vi "Teleop.vi"(10 "Match Info":T1={"Autonomous Elapsed Seconds"=0.0, "TeleOp Elapsed Seconds"=0.0, "Disabled Elapsed Seconds"=0.0, "Visited Autonomous"=FALSE, "Visited TeleOp"=FALSE, "Visited Disabled"=FALSE, "Autonomous Settings"={"Autonomous Style"=enum."Independent", "VI Refnum"=refnum}}, 11 "Call Context":T2) -> ()   [LabVIEW 2012]
doc: "This VI is called for each TeleOp packet received from the DS where the robot is not disabled. It is often used to read from the joysticks and update I/O or to update setpoints for timed control loops. It should complete and return within 20 milliseconds or it may miss DS packets."
uses:
  <vilib>/Rock Robotics/WPI/DriverStation/WPI_DriverStationDerivedRobotMode.ctl
  <vilib>/Rock Robotics/WPI/DriverStation/WPI_DriverStationMatch Info.ctl
  <vilib>/Rock Robotics/WPI/DriverStation/DriverStationLCD/WPI_DriverStationLCDLCDLine.ctl
  Robot Global Data.vi
  <vilib>/Rock Robotics/WPI/Joystick/WPI_JoystickGetSetRefNum.vi
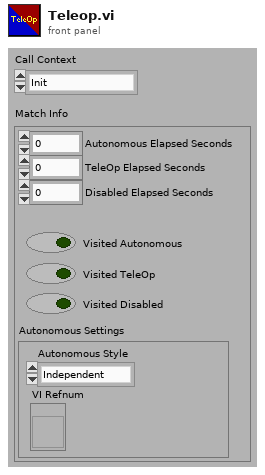
[diagram p1: front panel]
types:
  T1 = typedef "WPI_DriverStationMatch Info.ctl" = cluster{"Autonomous Elapsed Seconds":dbl, "TeleOp Elapsed Seconds":dbl, "Disabled Elapsed Seconds":dbl, "Visited Autonomous":bool, "Visited TeleOp":bool, "Visited Disabled":bool, "Autonomous Settings":cluster{"Autonomous Style":enum16{"Iterative", "Independent"}, "VI Refnum":refnum<vi>}}
  T2 = typedef "WPI_DriverStationDerivedRobotMode.ctl" = enum16{"Init", "Execute", "Stop"}
  T3 = typedef "WPI_DriverStationLCDLCDLine.ctl" = enum16{"Main - Line 1", "User - Line 2", "User - Line 3", "User - Line 4", "User - Line 5", "User - Line 6"}
  T4 = typedef "WPI_MotorControlDeviceRef.ctl" = cluster{"DeviceStatus":errorcluster, "Type":enum16{"PWM", "CAN"}, "PWM":cluster{"Digital Module":T5, "PWM Channel":T6, "DeadBand":T7}, "CAN":cluster{"Device Number":u8, "Control Mode":T8, "Semaphore":T9, "Max Vout":dbl}, "Invert":bool, "TransformRef":T10, "InvTransformRef":T10}
  T5 = typedef "FPGA_TypedefDigitalModule.ctl" = enum16{"Digital Module 1", "Digital Module 2"}
  T6 = typedef "FPGA_DIOPWMChannel.ctl" = enum8{"PWM 1", "PWM 2", "PWM 3", "PWM 4", "PWM 5", "PWM 6", "PWM 7", "PWM 8", "PWM 9", "PWM 10", "Invalid"}
  T7 = typedef "WPI_PWMDeadband.ctl" = cluster{"Name":string, "maxPositivePwm":i32, "minPositivePwm":i32, "centerPwm":i32, "maxNegativePwm":i32, "minNegativePwm":i32, "angularRange":u16}
  T8 = typedef "WPI_CANJaguar_ControlMode.ctl" = enum8{"Percent VBus", "Current", "Speed", "Position", "Voltage"}
  T9 = typedef "Semaphore RefNum" = refnum<k1>
  T10 = typedef "WPI_PWMTransform_ConPane.ctl" = refnum<vi>
  T11 = typedef "WPI_JoystickDevRef.ctl" = cluster{"Device":T12}
  T12 = typedef "WPI_JoystickDeviceEnum.ctl" = enum16{"USB 1", "USB 2", "USB 3", "USB 4", "Kinect 1", "Kinect 2"}
  T13 = typedef "WPI_JoystickButtonState.ctl" = cluster{"Button 1":bool, "Button 2":bool, "Button 3":bool, "Button 4":bool, "Button 5":bool, "Button 6":bool, "Button 7":bool, "Button 8":bool, "Button 9":bool, "Button 10":bool, "Button 11":bool, "Button 12":bool}
  T14 = cluster{"axis 1 (x)":dbl, "axis 2 (y)":dbl, "axis 3 (throttle)":dbl, "axis 4":dbl, "axis 5":dbl, "axis 6":dbl}
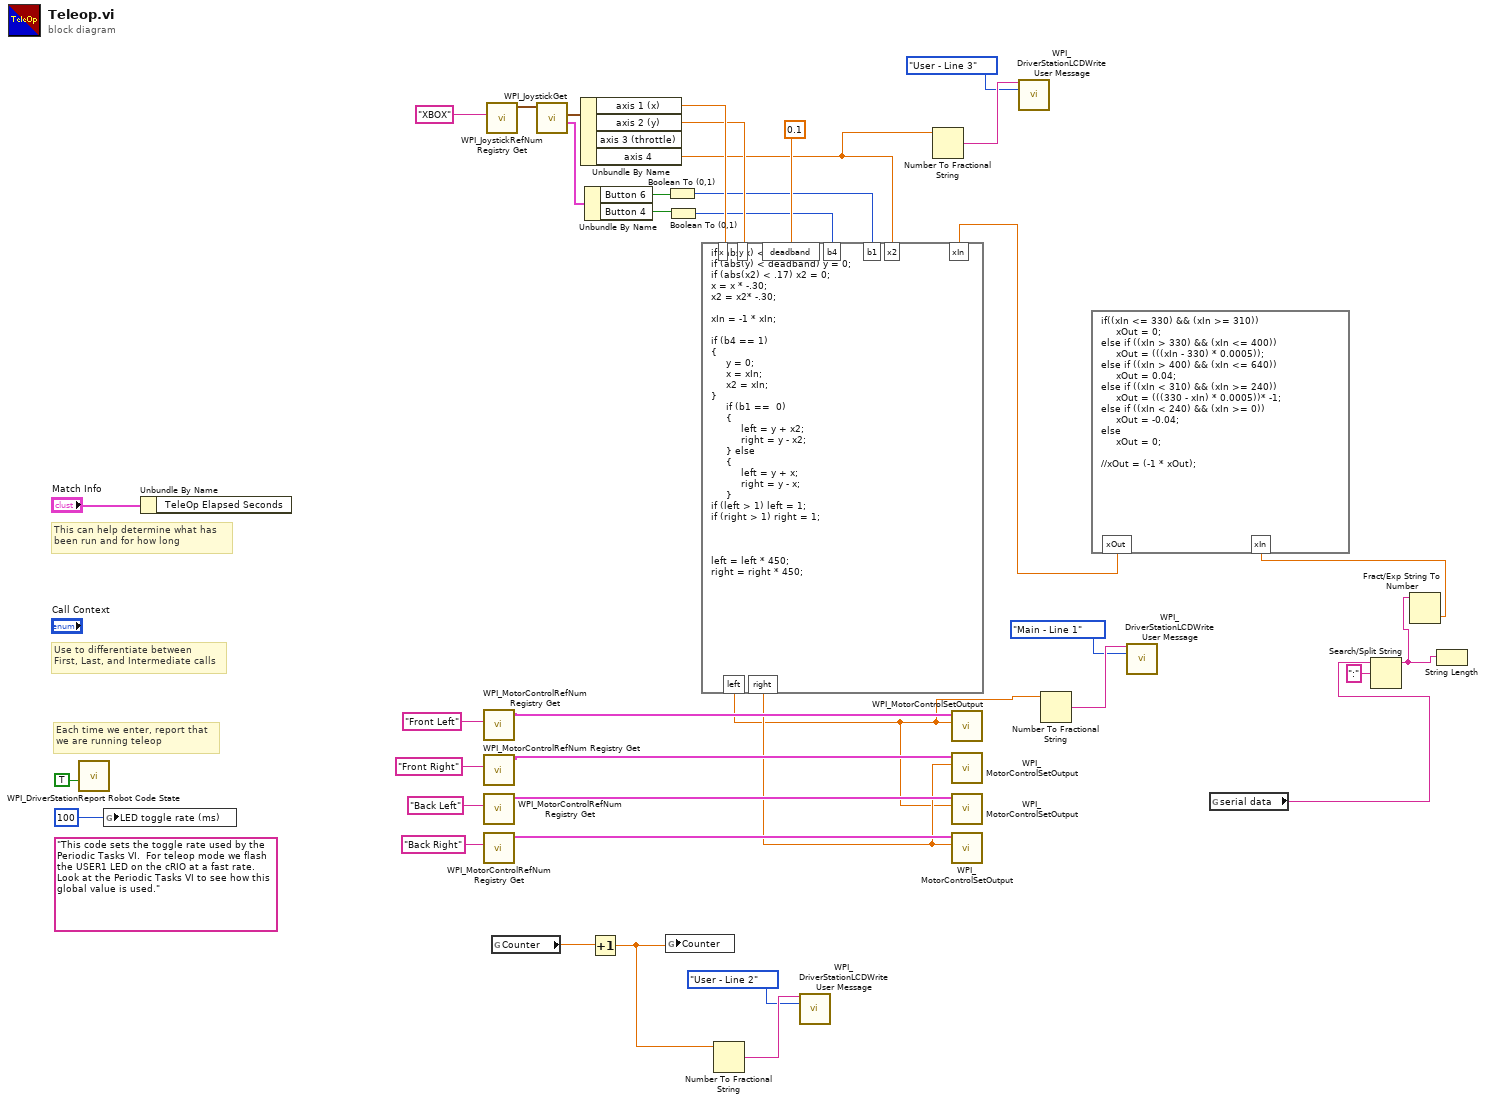
[diagram p0: block diagram]
diagram:
  (unwired) "This code sets the toggle rate used by the Periodic Tasks VI.  For teleop mode we flash the USER1 LED on the cRIO at a fast rate.  Look at the Periodic Tasks VI to see how this global value is used."
  # "Each time we enter, report that\nwe are running teleop"
  # "Use to differentiate between\nFirst, Last, and Intermediate calls"
  # "This can help determine what has\nbeen run and for how long"
  n1 = call <vilib>:"WPI_DriverStationReport Robot Code State.vi"("TeleOp"=TRUE ("Autonomous")) -> ()  [unwired: 10 in, 1 out]
  n2 = global write "Robot Global Data.vi" "LED toggle rate (ms)"(u32 100 ("LED ms toggle rate")) -> ()
  n3 = Unbundle By Name("Match Info") -> ()  [unwired: 1 out]
  n4 = call <vilib>:"WPI_MotorControlRefNum Registry Get.vi"("refnum name"="Front Left") -> ("MotorControlDevRef"=w30:T4)  [unwired: 9 in, 1 out]
  n5 = call <vilib>:"WPI_MotorControlRefNum Registry Get.vi"("refnum name"="Front Right") -> ("MotorControlDevRef"=w29:T4)  [unwired: 9 in, 1 out]
  n6 = call <vilib>:"WPI_MotorControlRefNum Registry Get.vi"("refnum name"="Back Left") -> ("MotorControlDevRef"=w28:T4)  [unwired: 9 in, 1 out]
  n7 = call <vilib>:"WPI_MotorControlRefNum Registry Get.vi"("refnum name"="Back Right") -> ("MotorControlDevRef"=w27:T4)  [unwired: 9 in, 1 out]
  n8 = call <vilib>:"WPI_JoystickRefNum Registry Get.vi"("refnum name"="XBOX") -> ("JoystickDevRef"=w24:T11)  [unwired: 1 in, 9 out]
  n9 = global read "Robot Global Data.vi" "Counter"() -> (w18:dbl)
  n10 = call <vilib>:"WPI_JoystickGet.vi"("JoystickDevRef"=w24) -> ("Buttons"=w11:T13, "Axes"=w23:T14)  [unwired: 1 in, 4 out]
  n11 = Unbundle By Name(w23) -> ("axis 1 (x)"=w22:dbl, "axis 2 (y)"=w12:dbl, "axis 4"=w8:dbl)  [unwired: 1 out]
  n12 = Unbundle By Name(w11) -> ("Button 6"=w10:bool, "Button 4"=w3:bool)
  n13 = Increment(x=w18) -> (x+1=w15:dbl)
  n14 = global write "Robot Global Data.vi" "Counter"(w15) -> ()
  n15 = Boolean To (0,1)(Boolean=w10) -> (0, 1=w9:i16)
  n16 = Boolean To (0,1)(Boolean=w3) -> (0, 1=w2:i16)
  n17 = Number To Fractional String(number=w15) -> (F-format string=w17:string)  [unwired: 3 in]
  n18 = call <vilib>:"WPI_DriverStationLCDWrite User Message.vi"("line text"=w17, "line"=WPI_DriverStationLCDLCDLine."User - Line 2") -> ()  [unwired: 13 in, 1 out]
  n19 = Number To Fractional String(number=w8) -> (F-format string=w14:string)  [unwired: 3 in]
  n20 = call <vilib>:"WPI_DriverStationLCDWrite User Message.vi"("line text"=w14, "line"=WPI_DriverStationLCDLCDLine."User - Line 3") -> ()  [unwired: 13 in, 1 out]
  n21 = global read "Robot Global Data.vi" "serial data"() -> (w1:string)
  n22 = Search/Split String(string=w1, search string/char (-)=":") -> (substring before match=w6:string)  [unwired: 1 in, 2 out]
  n23 = Fract/Exp String To Number(string=w6) -> (number=w5:dbl)  [unwired: 3 in, 1 out]
  n24 = formula code="if((xIn <= 330) && (xIn >= 310))\n     xOut = 0;\nelse if ((xIn > 330) && (xIn <= 400))\n     xOut = (((xIn - 330) * 0.0005));\nelse if ((xIn > 400) && (xIn <= 640))\n     xOut = 0.04;\nelse if ((xIn < 310) && (xIn >= 240))\n     xOut = (((330 - xIn) * 0.0005))* -1;\nelse if ((xIn < 240) && (xIn >= 0))\n     xOut = -0.04;\nelse\n     xOut = 0;\n\n//xOut = (-1 * xOut);"("xIn"=w5) -> ("xOut"=w4:dbl)
  n25 = formula code="if (abs(x) < .17) x = 0;\nif (abs(y) < deadband) y = 0;\nif (abs(x2) < .17) x2 = 0;\nx = x * -.30;\nx2 = x2* -.30;\n\nxIn = -1 * xIn;\n\nif (b4 == 1)\n{\n     y = 0;\n     x = xIn;\n     x2 = xIn;\n}\n     if (b1 ==  0)\n     {\n          left = y + x2;\n          right = y - x2;\n     } else\n     {\n          left = y + x;\n          right = y - x;\n     }\nif (left > 1) left = 1;\nif (right > 1) right = 1;\n\n\n\nleft = left * 450;\nright = right * 450;"("x"=w22, "y"=w12, "deadband"=0.1 ("input variable"), "b1"=w9, "x2"=w8, "xIn"=w4, "b4"=w2) -> ("left"=w21:dbl, "right"=w26:dbl)
  n26 = call <vilib>:"WPI_MotorControlSetOutput.vi"("Output"=w21, "MotorControlDevRef"=w30) -> ()  [unwired: 7 in, 3 out]
  n27 = call <vilib>:"WPI_MotorControlSetOutput.vi"("Output"=w26, "MotorControlDevRef"=w29) -> ()  [unwired: 7 in, 3 out]
  n28 = call <vilib>:"WPI_MotorControlSetOutput.vi"("Output"=w21, "MotorControlDevRef"=w28) -> ()  [unwired: 7 in, 3 out]
  n29 = call <vilib>:"WPI_MotorControlSetOutput.vi"("Output"=w26, "MotorControlDevRef"=w27) -> ()  [unwired: 7 in, 3 out]
  n30 = Number To Fractional String(number=w21) -> (F-format string=w20:string)  [unwired: 3 in]
  n31 = call <vilib>:"WPI_DriverStationLCDWrite User Message.vi"("line text"=w20, "line"=WPI_DriverStationLCDLCDLine."Main - Line 1") -> ()  [unwired: 13 in, 1 out]
  n32 = String Length(string=w6) -> ()  [unwired: 1 out]
